vi "check and clear serial port.vi"(8 "error in (no error)":errorcluster, 9 "expected Number of Bytes at Serial Port (default: 0)":u32, 10 "timeout (default: 100ms)":i32=100 min=100 max=1000 step=10, 11 "VISA resource name in":refnum<visa-resource-name>) -> (0 "error out":errorcluster, 1 "read buffer":string, 2 "number of bytes actually read":u32, 3 "VISA resource name out":refnum<visa-resource-name>)   [LabVIEW 2012]
doc: "SciScan 1.2 160622"
uses:
  <vilib>/Platform/TimedLoop/XDataNode/timing_clust.ctl
  <vilib>/Platform/TimedLoop/XDataNode/nitl_modes.ctl
  <vilib>/Platform/TimedLoop/XDataNode/wakeup.ctl
  <vilib>/Platform/TimedLoop/XDataNode/XDataNode.xnode
  <vilib>/Platform/TimedLoop/XDataNode/XDNodeRunTimeDep.lvlib
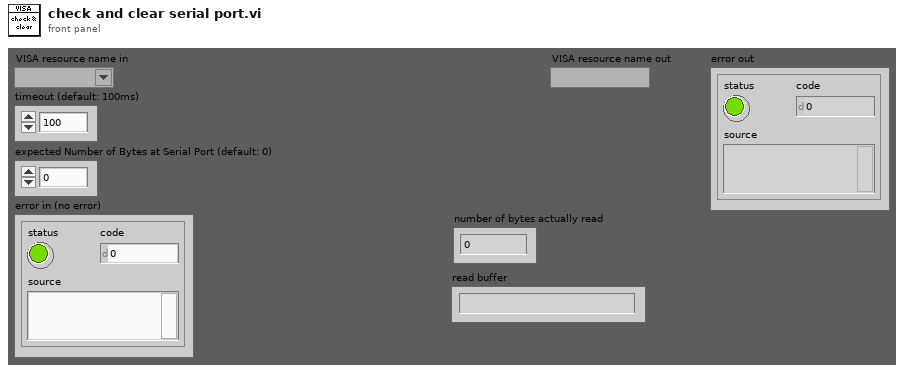
[diagram p1: front panel]
types:
  T1 = typedef "XDNodeRunTimeDep.lvlib/timing_clust.ctl" = cluster{"Expected End [f-1]":u64, "Actual End [f-1]":u64, "Finished Late? [f-1]":bool, "Expected End [i-1]":u64, "Actual End [i-1]":u64, "Finished Late? [i-1]":bool, "Expected Start [i]":u64, "Actual Start [i]":u64, "Expected Start [f]":u64, "Actual Start [f]":u64, "Source Name":string, "Structure Name":string, "Period":i64, "Deadline":i64, "Offset":i64, "Start":i64, "Priority":i32, "Timeout":i32, "Mode":T2, "Wakeup Reason":T3, "Error":errorcluster, "Source Type":string, "Secondary Source Type":string, "Global End Time":u64, "Global Start Time":u64, "Frame Duration":u64, "Iteration Duration":u64, "Assigned CPU":i32, "I/O Scan Engine Mode":u32}
  T2 = typedef "XDNodeRunTimeDep.lvlib/nitl_modes.ctl" = enum32{"No Change", "Process missed periods, maintain original phase", "Discard missed periods, maintain original phase", "Process missed periods, ignore original phase", "Discard missed periods, ignore original phase"}
  T3 = typedef "XDNodeRunTimeDep.lvlib/wakeup.ctl" = enum32{"Normal", "Aborted", "Asynchronous wakeup", "Timing source error", "Timed loop error", "Timeout"}
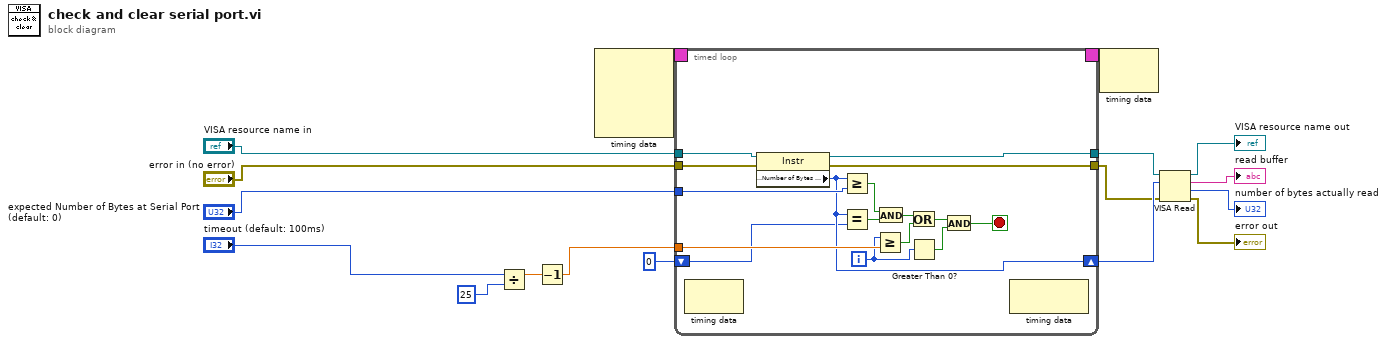
[diagram p0: block diagram]
diagram:
  n1 = Divide(x="timeout (default: 100ms)", y=25) -> (x/y=w13:dbl)
  n2 = Decrement(x=w13) -> (x-1=w10:dbl)
  n3 = node-c288() -> (w17:T1)  [unwired: 4 in]
  n4 = timed-loop {
    timing: w17 -> [_]
    timing-out: [_] -> w16
    tunnel: "VISA resource name in" -> [w33]
    tunnel: [w31] -> w8
    tunnel: w10 -> [w30]
    tunnel: "expected Number of Bytes at Serial Port (default: 0)" -> [w29]
    tunnel: "error in (no error)" -> [w26]
    tunnel: [w25] -> w3
    shift-right: [w20] -> w9
    shift-left: u32 0 ("Bytes at Port") -> [w19]
    i -> [w22]
    stop <- w24 stop-if-true
    n5 = node-c288() -> ()  [unwired: 1 in, 1 out]
    n6 = property class="Instr"(reference=w33, error in=w26) -> (reference out=w31:refnum<visa-resource-name>, error out=w25:errorcluster, "Serial Settings:Number of Bytes at Serial Port"=w20:u32)
    n7 = Greater Or Equal?(x=w20, y=w29) -> (x >= y?=w27:bool)
    n8 = Equal?(x=w20, y=w19) -> (x = y?=w18:bool)
    n9 = Greater Or Equal?(x=w22, y=w30) -> (x >= y?=w32:bool)
    n10 = And(x=w27, y=w18) -> (x .and. y?=w21:bool)
    n11 = Or(x=w21, y=w32) -> (x .or. y?=w28:bool)
    n12 = Greater Than 0?(x=w22) -> (x > 0?=w23:bool)
    n13 = And(x=w28, y=w23) -> (x .and. y?=w24:bool)
    n14 = node-c288() -> ()  [unwired: 1 in, 1 out]
  }
  n15 = node-c288(w16) -> ()  [unwired: 1 out]
  n16 = VISA Read(VISA resource name=w8, byte count=w9, error in (no error)=w3) -> (VISA resource name out=→"VISA resource name out":refnum<visa-resource-name>, read buffer=→"read buffer":string, return count=→"number of bytes actually read":u32, error out=→"error out":errorcluster)
